vi "OE1022D_Read 1 parameter_stable.vi"(1 "数据转换":u8[](array[numeric]), 5 "Parameter 3":u16(ring) items=["AUX1", "AUX2", "AUX3", "AUX4"], 7 "Parameter 2":u16(ring) items=["X", "Y", "R", "Theta", "Frequency", "Noise", "Xh1", "Yh1", "Rh1", "Theta h1", "Xh2", "Yh2", "Rh2", "Theta h2"], 8 "错误输入（无错误）":errorcluster, 9 "Parameter":u16(ring) items=["X", "Y", "R", "Theta", "Frequency", "Noise", "Xh1", "Yh1", "Rh1", "Theta h1", "Xh2", "Yh2", "Rh2", "Theta h2"], 10 "Channel (0: A)":u16(ring) items=["Channel A", "Channel B", "ADC"], 11 "VISA resource name":refnum<visa-resource-name>) -> (0 "error out":errorcluster, 2 "Measurement":dbl format="%.3p", 3 "VISA resource name out":refnum<visa-resource-name>)   [LabVIEW 2021]
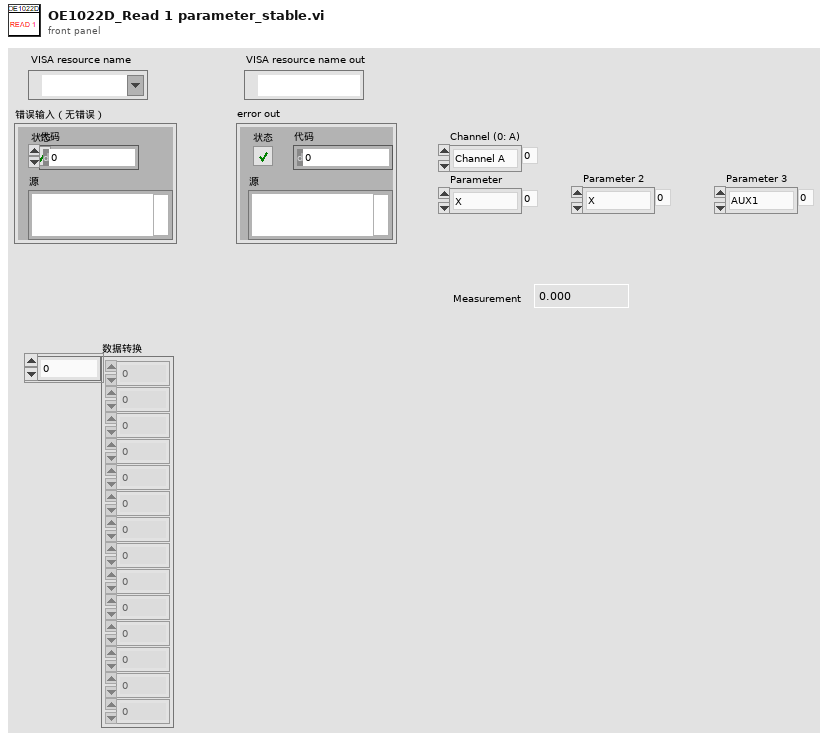
[diagram p1: front panel]
types:
  T1 = cluster{"AD1":dbl[], "AD2":dbl[], "AD3":dbl[], "AD4":dbl[]}
  T2 = cluster{"XA":dbl[], "YA":dbl[], "FrequencyA":dbl[], "NoiseA":dbl[], "Xh1A":dbl[], "Yh1A":dbl[], "Xh2A":dbl[], "Yh2A":dbl[]}
  T3 = cluster{"XB":dbl[], "YB":dbl[], "FrequencyB":dbl[], "NoiseB":dbl[], "Xh1B":dbl[], "Yh1B":dbl[], "Xh2B":dbl[], "Yh2B":dbl[], "Xh2B":dbl[]}
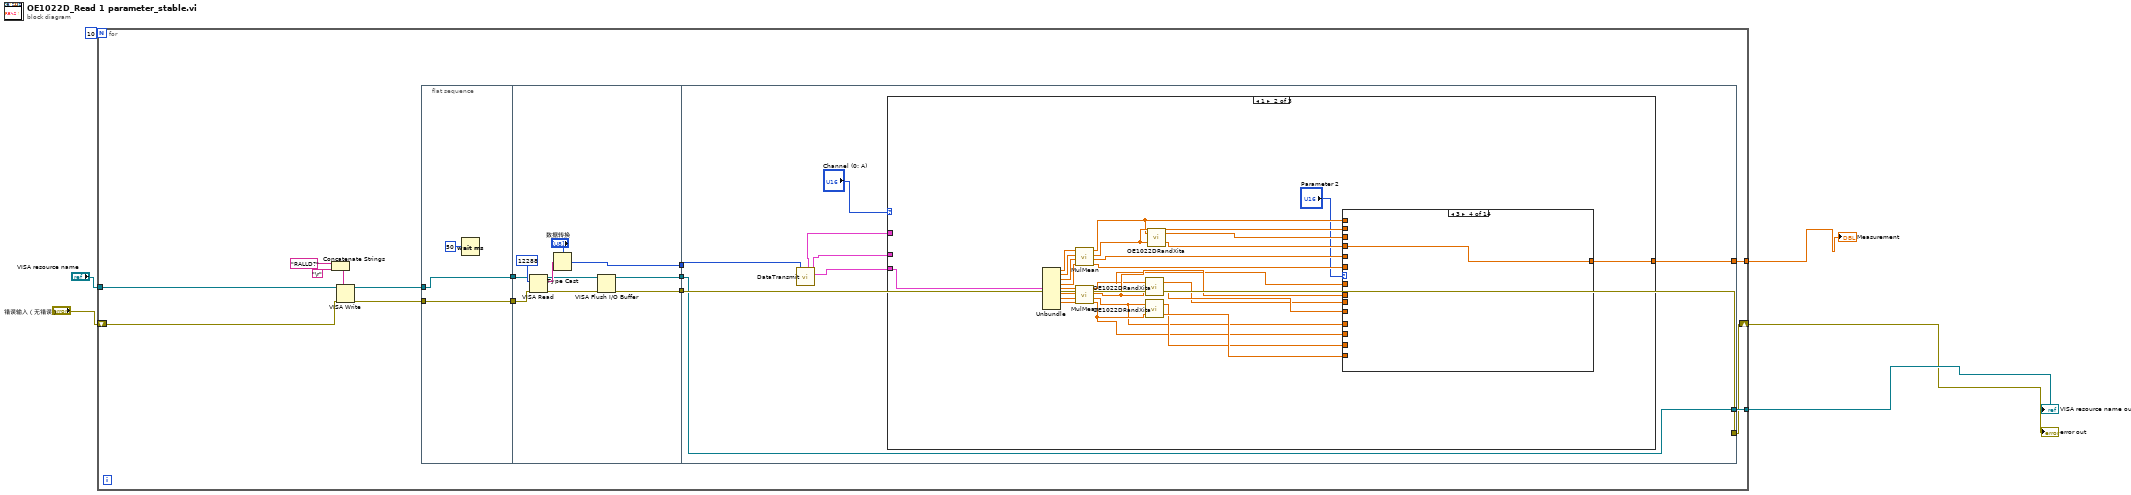
[diagram p0: block diagram]
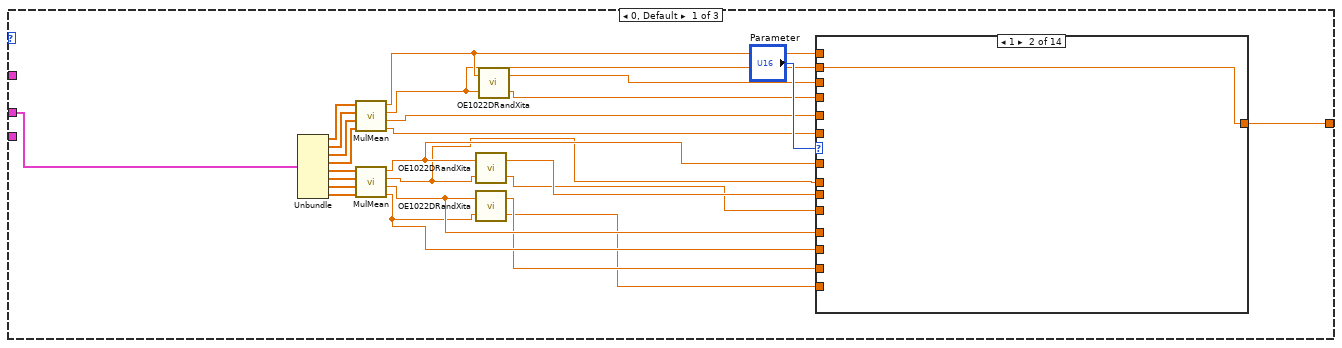
[diagram p2: hidden frame]
diagram:
  n1 = for {
    N: 10 -> [_]
    tunnel: [w11] -> w6
    shift-right: [w10] -> w5
    shift-left: "错误输入（无错误）" -> [w7]
    tunnel: [w9] -> w1
    tunnel: "VISA resource name" -> [w8]
    n2 = Concatenate Strings("RALLD?" ("命令输入"), "\r") -> (w15:string)
    n3 = VISA Write(VISA resource name=w8, write buffer=w15, error in (no error)=w7) -> (VISA resource name out=w13:refnum<visa-resource-name>, error out=w12:errorcluster)  [unwired: 1 out]
    n4 = flat-sequence {
      tunnel: w13 -> [w22]
      tunnel: w12 -> [w23]
      tunnel: [w23] -> w21
      tunnel: [w22] -> w20
      tunnel: w21 -> [w26]
      tunnel: w20 -> [w25]
      tunnel: [w29] -> w19
      tunnel: [w28] -> w18
      tunnel: [w27] -> w17
      tunnel: w19 -> [w39]
      tunnel: w18 -> [w41]
      tunnel: w17 -> [w40]
      tunnel: [w41] -> w10
      tunnel: [w40] -> w11
      tunnel: [w35] -> w9
      frame #0 {
        n5 = Wait (ms)(milliseconds to wait=u32 50 ("等待时间（毫秒）")) -> ()  [unwired: 1 out]
      }
      frame #1 {
        n6 = VISA Read(VISA resource name=w25, byte count=12288, error in (no error)=w26) -> (VISA resource name out=w31:refnum<visa-resource-name>, read buffer=w33:string, error out=w32:errorcluster)  [unwired: 1 out]
        n7 = Type Cast(type="数据转换", x=w33) -> (*(type *) &x=w29:u8[])
        n8 = VISA Flush I/O Buffer(VISA resource name=w31, error in (no error)=w32) -> (VISA resource name out=w27:refnum<visa-resource-name>, error out=w28:errorcluster)  [unwired: 1 in]
      }
      frame #2 {
        n9 = call <instrlib>:"DataTransmit.vi"("数据输入"=w39) -> ("输出簇ADC"=w38:T1, "输出簇A"=w37:T2, "输出簇B"=w36:T3)  [unwired: 2 in, 2 out]
        n10 = case shown="1" "Channel (0: A)" {
          tunnel: w38 -> [_ _ w127]
          tunnel: w37 -> [w58 _ _]
          tunnel: w36 -> [_ w82 _]
          tunnel: [w53 w83 w121] -> w35
          frame 0, Default {
            n11 = Unbundle(w58) -> ("XA"=w59:dbl[], "YA"=w60:dbl[], "FrequencyA"=w61:dbl[], "NoiseA"=w62:dbl[], "Xh1A"=w63:dbl[], "Yh1A"=w64:dbl[], "Xh2A"=w65:dbl[], "Yh2A"=w66:dbl[])
            n12 = call <instrlib>:"MulMean.vi"("IN 4"=w62, "IN 3"=w61, "IN 2"=w60, "IN 1"=w59) -> ("mean 4"=w47:dbl, "mean 3"=w48:dbl, "mean 2"=w56:dbl, "mean 1"=w57:dbl)  [unwired: 4 in]
            n13 = call <instrlib>:"MulMean.vi"("IN 4"=w66, "IN 3"=w65, "IN 2"=w64, "IN 1"=w63) -> ("mean 4"=w45:dbl, "mean 3"=w46:dbl, "mean 2"=w51:dbl, "mean 1"=w52:dbl)  [unwired: 4 in]
            n14 = call <instrlib>:"OE1022DRandXita.vi"("Y"=w51, "X"=w52) -> ("θ (°)"=w49:dbl, "R"=w50:dbl)
            n15 = call <instrlib>:"OE1022DRandXita.vi"("Y"=w45, "X"=w46) -> ("θ (°)"=w43:dbl, "R"=w44:dbl)
            n16 = call <instrlib>:"OE1022DRandXita.vi"("Y"=w56, "X"=w57) -> ("θ (°)"=w54:dbl, "R"=w55:dbl)
            n17 = case shown="1" "Parameter" {
              tunnel: w57 -> [w68 _ _ _ _ _ _ _ _ _ _ _ _ _]
              tunnel: w56 -> [_ w69 _ _ _ _ _ _ _ _ _ _ _ _]
              tunnel: w55 -> [_ _ w70 _ _ _ _ _ _ _ _ _ _ _]
              tunnel: w54 -> [_ _ _ w71 _ _ _ _ _ _ _ _ _ _]
              tunnel: [w68 w69 w70 w71 w72 w73 w74 w75 w76 w77 w78 w79 w80 w81] -> w53
              tunnel: w52 -> [_ _ _ _ _ _ w74 _ _ _ _ _ _ _]
              tunnel: w51 -> [_ _ _ _ _ _ _ w75 _ _ _ _ _ _]
              tunnel: w50 -> [_ _ _ _ _ _ _ _ w76 _ _ _ _ _]
              tunnel: w49 -> [_ _ _ _ _ _ _ _ _ w77 _ _ _ _]
              tunnel: w48 -> [_ _ _ _ w72 _ _ _ _ _ _ _ _ _]
              tunnel: w47 -> [_ _ _ _ _ w73 _ _ _ _ _ _ _ _]
              tunnel: w46 -> [_ _ _ _ _ _ _ _ _ _ w78 _ _ _]
              tunnel: w45 -> [_ _ _ _ _ _ _ _ _ _ _ w79 _ _]
              tunnel: w44 -> [_ _ _ _ _ _ _ _ _ _ _ _ w80 _]
              tunnel: w43 -> [_ _ _ _ _ _ _ _ _ _ _ _ _ w81]
              frame 0, Default {
              }
              frame 1 {
              }
              frame 2 {
              }
              frame 3 {
              }
              frame 4 {
              }
              frame 5 {
              }
              frame 6 {
              }
              frame 7 {
              }
              frame 8 {
              }
              frame 9 {
              }
              frame 10 {
              }
              frame 11 {
              }
              frame 12 {
              }
              frame 13 {
              }
            }
          }
          frame 1 {
            n18 = Unbundle(w82) -> ("XB"=w92:dbl[], "YB"=w91:dbl[], "FrequencyB"=w90:dbl[], "NoiseB"=w89:dbl[], "Xh1B"=w88:dbl[], "Yh1B"=w87:dbl[], "Xh2B"=w86:dbl[], "Yh2B"=w85:dbl[])  [unwired: 1 out]
            n19 = call <instrlib>:"MulMean.vi"("IN 4"=w89, "IN 3"=w90, "IN 2"=w91, "IN 1"=w92) -> ("mean 4"=w102:dbl, "mean 3"=w101:dbl, "mean 2"=w94:dbl, "mean 1"=w93:dbl)  [unwired: 4 in]
            n20 = call <instrlib>:"MulMean.vi"("IN 4"=w85, "IN 3"=w86, "IN 2"=w87, "IN 1"=w88) -> ("mean 4"=w104:dbl, "mean 3"=w103:dbl, "mean 2"=w98:dbl, "mean 1"=w97:dbl)  [unwired: 4 in]
            n21 = call <instrlib>:"OE1022DRandXita.vi"("Y"=w98, "X"=w97) -> ("θ (°)"=w100:dbl, "R"=w99:dbl)
            n22 = call <instrlib>:"OE1022DRandXita.vi"("Y"=w104, "X"=w103) -> ("θ (°)"=w106:dbl, "R"=w105:dbl)
            n23 = call <instrlib>:"OE1022DRandXita.vi"("Y"=w94, "X"=w93) -> ("θ (°)"=w96:dbl, "R"=w95:dbl)
            n24 = case shown="3" "Parameter 2" {
              tunnel: w93 -> [w107 _ _ _ _ _ _ _ _ _ _ _ _ _]
              tunnel: w94 -> [_ w108 _ _ _ _ _ _ _ _ _ _ _ _]
              tunnel: w95 -> [_ _ w109 _ _ _ _ _ _ _ _ _ _ _]
              tunnel: w96 -> [_ _ _ w110 _ _ _ _ _ _ _ _ _ _]
              tunnel: [w107 w108 w109 w110 w111 w112 w113 w114 w115 w116 w117 w118 w119 w120] -> w83
              tunnel: w97 -> [_ _ _ _ _ _ w113 _ _ _ _ _ _ _]
              tunnel: w98 -> [_ _ _ _ _ _ _ w114 _ _ _ _ _ _]
              tunnel: w99 -> [_ _ _ _ _ _ _ _ w115 _ _ _ _ _]
              tunnel: w100 -> [_ _ _ _ _ _ _ _ _ w116 _ _ _ _]
              tunnel: w101 -> [_ _ _ _ w111 _ _ _ _ _ _ _ _ _]
              tunnel: w102 -> [_ _ _ _ _ w112 _ _ _ _ _ _ _ _]
              tunnel: w103 -> [_ _ _ _ _ _ _ _ _ _ w117 _ _ _]
              tunnel: w104 -> [_ _ _ _ _ _ _ _ _ _ _ w118 _ _]
              tunnel: w105 -> [_ _ _ _ _ _ _ _ _ _ _ _ w119 _]
              tunnel: w106 -> [_ _ _ _ _ _ _ _ _ _ _ _ _ w120]
              frame 0, Default {
              }
              frame 1 {
              }
              frame 2 {
              }
              frame 3 {
              }
              frame 4 {
              }
              frame 5 {
              }
              frame 6 {
              }
              frame 7 {
              }
              frame 8 {
              }
              frame 9 {
              }
              frame 10 {
              }
              frame 11 {
              }
              frame 12 {
              }
              frame 13 {
              }
            }
          }
          frame 2 {
            n25 = Unbundle By Name(w127) -> ("AD1"=w131:dbl[], "AD2"=w130:dbl[], "AD3"=w129:dbl[], "AD4"=w128:dbl[])
            n26 = call <instrlib>:"MulMean.vi"("IN 4"=w128, "IN 3"=w129, "IN 2"=w130, "IN 1"=w131) -> ("mean 4"=w122:dbl, "mean 3"=w123:dbl, "mean 2"=w124:dbl, "mean 1"=w125:dbl)  [unwired: 4 in]
            n27 = case shown="0, Default" "Parameter 3" {
              tunnel: w125 -> [w132 _ _ _]
              tunnel: w124 -> [_ w133 _ _]
              tunnel: w123 -> [_ _ w134 _]
              tunnel: w122 -> [_ _ _ w135]
              tunnel: [w132 w133 w134 w135] -> w121
              frame 0, Default {
              }
              frame 1 {
              }
              frame 2 {
              }
              frame 3 {
              }
            }
          }
        }
      }
    }
  }
  "VISA resource name out" <- w6
  "error out" <- w5
  "Measurement" <- w1
